vi "fgv_Send-Serial.vi"(7 "cmd":enum16{"init", "read", "write", "close"}(ring), 8 "error in":errorcluster, 11 "write buff":string) -> (0 "error out":errorcluster, 2 "byte n":u32(graph), 3 "read_buffer":string)   [LabVIEW 2019]
uses:
  Ctrl/cmd_common.ctl
  <vilib>/Instr/_visa.llb/VISA Configure Serial Port (Instr).vi
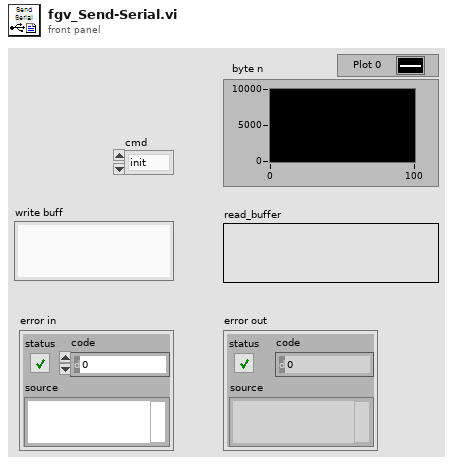
[diagram p1: front panel]
types:
  T1 = typedef "cmd_common.ctl" = enum16{"read", "write"}
  T2 = typedef "GNSS-Ntrip config.ctl" = cluster{"Current NtripClient Account":cluster{"id":string, "pwd":string, "ref pt":string, "address":string, "port ":u16}, "Mount points":u16, "Ref r size":dbl, "TMarr limit":i32, "Sel NMEA type":enum16{"$GPGSV", "$GLGSV", "$GPGGA", "$GAGSV", "$GBGSV", "$GNGLL", "$GNGGA", "$GNGSA", "$GNRMC", "$GNVTG"}, "Local Time offset":u32, "Write delay ms":u32, "GNSS Serial delay":u32, "Extra Serial delay":u32, "Ntrip accounts":cluster{"id":string, "pwd":string, "ref pt":string, "address":string, "port ":u16}[], "Send Serial config":cluster{"NMEA out port":refnum<visa-resource-name>, "baud rate":u32}}
  T3 = typedef "gnss_config-2.ctl" = cluster{"Port":refnum<visa-resource-name>, "rate":u32}
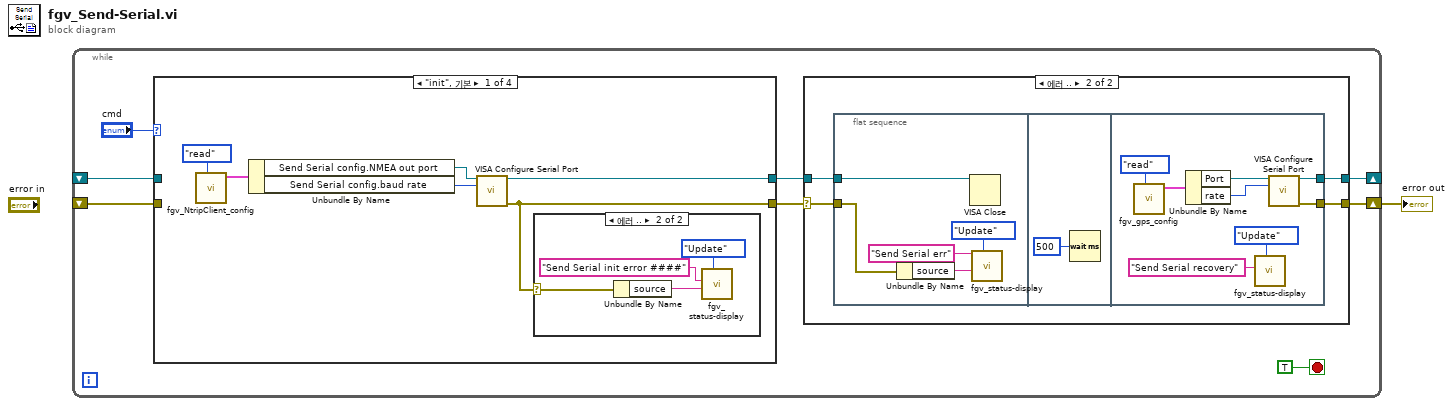
[diagram p0: block diagram]
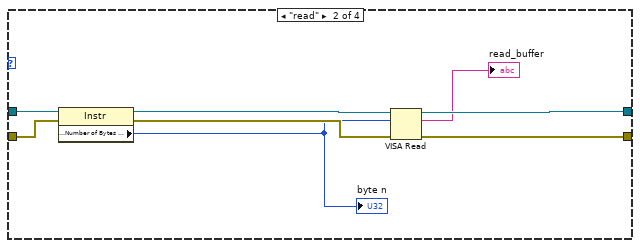
[diagram p4: hidden frame]
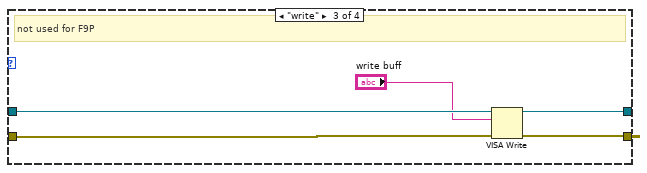
[diagram p5: hidden frame]
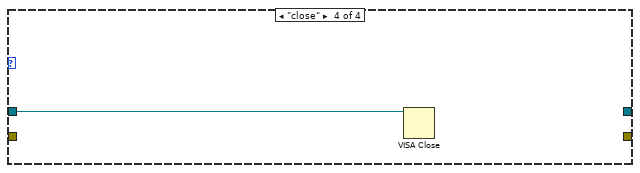
[diagram p6: hidden frame]
diagram:
  n1 = while {
    shift-right: [w2] -> _
    shift-left: _ -> [w7]
    shift-right: [w3] -> w1
    shift-left: _ -> [w6]
    stop <- TRUE stop-if-true
    n2 = case shown="\"init\", 기본" "cmd" {
      tunnel: [w35 w45 w50 _] -> w4
      tunnel: [w34 w44 w49 _] -> w5
      tunnel: w7 -> [_ w47 w51 w53]
      tunnel: w6 -> [_ w42 w52 _]
      frame "init", Default {
        n3 = call "fgv_NtripClient_config.vi"("cmd"=cmd_common."read") -> ("config val out"=w32:T2)  [unwired: 10 in]
        n4 = Unbundle By Name(w32) -> ("Send Serial config.NMEA out port"=w30:refnum<visa-resource-name>, "Send Serial config.baud rate"=w31:u32)
        n5 = call-poly "VISA Configure Serial Port"("VISA resource name"=w30, "baud rate (9600)"=w31) -> ("VISA resource name out"=w35:refnum<visa-resource-name>, "error out"=w34:errorcluster)  [unwired: 12 in]
        n6 = case shown="에러 .." w34 {
          selector: w34 -> [_ w38]
          frame No Error {
          }
          frame Error {
            n7 = Unbundle By Name(w38) -> ("source"=w37:string)
            n8 = call "fgv_status-display.vi"("Mode"=enum16{"Initial", "Update", "Clear"}."Update", "detail"=w37, "title"="Send Serial init error ####" ("String in")) -> ()  [unwired: 8 in, 1 out]
          }
        }
      }
      frame "read" {
        n9 = property class="Instr"(reference=w47, error in=w42) -> (reference out=w46:refnum<visa-resource-name>, error out=w43:errorcluster, "Serial Settings:Number of Bytes at Serial Port"=w40:u32)
        "byte n" <- w40
        n10 = VISA Read(VISA resource name=w46, byte count=w40, error in (no error)=w43) -> (VISA resource name out=w45:refnum<visa-resource-name>, read buffer=→"read_buffer":string, error out=w44:errorcluster)  [unwired: 1 out]
      }
      frame "write" {
        # "not used for F9P"
        n11 = VISA Write(VISA resource name=w51, write buffer="write buff", error in (no error)=w52) -> (VISA resource name out=w50:refnum<visa-resource-name>, error out=w49:errorcluster)  [unwired: 1 out]
      }
      frame "close" {
        n12 = VISA Close(VISA resource name=w53) -> ()  [unwired: 1 in, 1 out]
      }
    }
    n13 = case shown="에러 .." w5 {
      selector: w5 -> [w10 w12]
      tunnel: w4 -> [w11 w15]
      tunnel: [w10 w14] -> w3
      tunnel: [w11 w13] -> w2
      frame No Error {
      }
      frame Error {
        n14 = flat-sequence {
          tunnel: w15 -> [w20]
          tunnel: w12 -> [w18]
          tunnel: [w25] -> w14
          tunnel: [w24] -> w13
          frame #0 {
            n15 = Unbundle By Name(w18) -> ("source"=w17:string)
            n16 = VISA Close(VISA resource name=w20) -> ()  [unwired: 1 in, 1 out]
            n17 = call "fgv_status-display.vi"("Mode"=enum16{"Initial", "Update", "Clear"}."Update", "detail"=w17, "title"="Send Serial err") -> ()  [unwired: 8 in, 1 out]
          }
          frame #1 {
            n18 = Wait (ms)(milliseconds to wait=u32 500) -> ()  [unwired: 1 out]
          }
          frame #2 {
            n19 = call "fgv_gps_config.vi"("cmd"=enum16{"read", "write"}."read") -> ("GNSS cfg out"=w29:T3)  [unwired: 9 in, 1 out]
            n20 = Unbundle By Name(w29) -> ("Port"=w26:refnum<visa-resource-name>, "rate"=w27:u32)
            n21 = call "fgv_status-display.vi"("Mode"=enum16{"Initial", "Update", "Clear"}."Update", "title"="Send Serial recovery" ("String in 1")) -> ()  [unwired: 9 in, 1 out]
            n22 = call-poly "VISA Configure Serial Port"("VISA resource name"=w26, "baud rate (9600)"=w27) -> ("VISA resource name out"=w24:refnum<visa-resource-name>, "error out"=w25:errorcluster)  [unwired: 12 in]
          }
        }
      }
    }
  }
  "error out" <- w1
